vi "LCP Get Syringe Param.vi"(8 "error in (no error)":errorcluster caption="Fehler (Eingang, kein Fehler)", 11 "Pump Handle":i64) -> (0 "error out":errorcluster caption="Fehler (Ausgang)", 2 "Maximum Piston Stroke (mm)":dbl, 3 "Inner Diameter (mm)":dbl)   [LabVIEW 2023, in "labbCAN_Pump_API.lvlib"]
doc: "LCP_Func long LCP_CALL LCP_GetSyringeParam(dev_hdl hPump,\n double *pInnerDiameter_mm,\n double *pMaxPistonStroke_mm);"
uses:
  labbCAN_Pump_API.lvlib
  labbCAN_Pump_API.dll
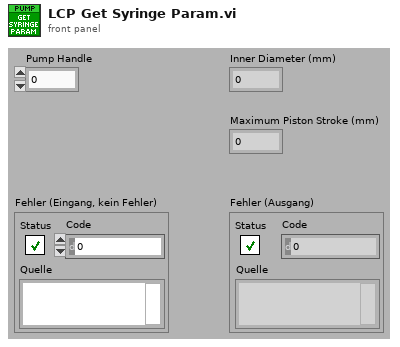
[diagram p1: front panel]
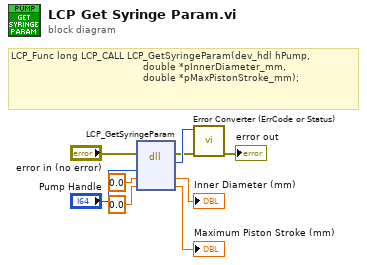
[diagram p0: block diagram]
diagram:
  # "LCP_Func long LCP_CALL LCP_GetSyringeParam(dev_hdl hPump,\n                                            double *pInnerDiameter_mm,\n                                            double *pMaxPistonStroke_mm);"
  n1 = dll-call lib="C:/GIT/DensityGradientProject/CETONI_SDK/labbCAN_Pump_API.*" fn="LCP_GetSyringeParam"(error in="error in (no error)", "hPump"="Pump Handle", "pInnerDiameter_mm"=0.0, "pMaxPistonStroke_mm"=0.0) -> (error out=w2:errorcluster, "Rückgabetyp"=w3:i32, "pInnerDiameter_mm"=→"Inner Diameter (mm)":dbl, "pMaxPistonStroke_mm"=→"Maximum Piston Stroke (mm)":dbl)  [unwired: 3 in, 1 out]
  n2 = call "Error Converter (ErrCode or Status).vi"("error in (no error)"=w2, "error code"=w3) -> ("error out"=→"error out":errorcluster)  [unwired: 9 in]
